vi "PostLoop.vi"(6 "Error":errorcluster, 7 "Actor":refnum<class "Actor.lvclass">) -> (5 "Actor":refnum<class "Actor.lvclass">)   [LabVIEW 2020, in "_Template.lvlib" / "{{Actor}}.lvlib" / "Actor.lvclass"]
uses:
  Actor.lvclass
  Actor.lvclass/Actor.ctl
  jettl/jettl/Actor/Actor.lvclass
panel:
  # "This front panel should not be manipulated."
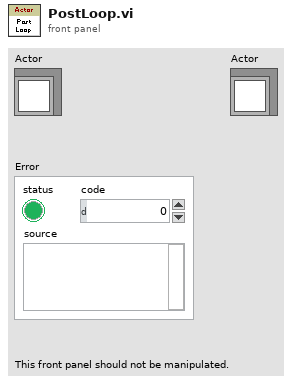
[diagram p1: front panel]
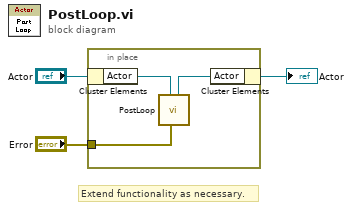
[diagram p0: block diagram]
diagram:
  # "Extend functionality as necessary."
  n1 = in-place {
    in-place-border: "Error" -> [w4]
    n2 = in-place-cluster #1("Actor") -> ("Actor"=w6:refnum<class "Actor.lvclass">)
    n3 = call-dynamic "PostLoop.vi"("Error"=w4, "Actor"=w6) -> ("Actor"=w5:refnum<class "Actor.lvclass">)  [unwired: 9 in]
    n4 = in-place-cluster #1("Actor"=w5) -> (→"Actor":refnum<class "Actor.lvclass">)
  }
